vi "User Interface Global.vi"(6 "data2":variant, 7 "command (Update UI)":T2=enum."Update UI", 8 "error in":errorcluster, 9 "data1":variant, 10 "action":T1, 11 "user interface queue reference":T3) -> (0 "error out":errorcluster)   [LabVIEW 2011]
uses:
  Controls/User Interface Queue Reference.ctl
  Controls/User Interface Control.ctl
  Controls/User Interface Action.ctl
  User Interface Global.ctl
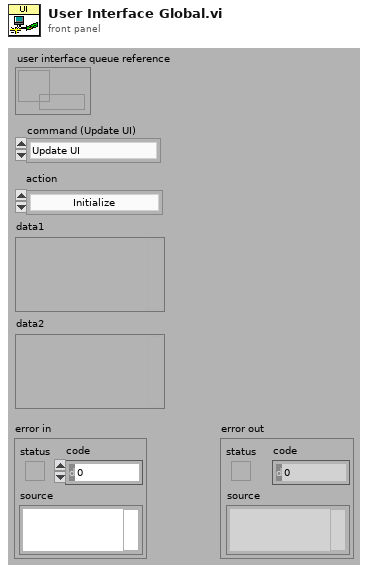
[diagram p1: front panel]
types:
  T1 = typedef "User Interface Action.ctl" = enum16{"Initialize", "Data Acquisition Disable", "Data View Disable", "Sample Set", "Sample Set 2D Data", "Sample Set x0 & dx", "Sample Add", "Sample Set Cursor", "Sample Set Offset & Multiplier", "Sample Set Axis Labels", "Sample Parameters Disabled", "Sample Parameters Update", "Run Update", "Run Set Offset & Multiplier", "Run Set Axis Labels", "Run Set Cursor", "Run Set Disabled", "Run Parameters Update", "Run Parameters Disabled", "Run Number Set", "Run Number Set Range", "Run Number Set Disabled", "Sample Number Set", "Sample Number Set Range", "Notes Set Value", "Update Plot", "Set Plot Parameters", "Update Concentration Plot", "Time Set", "Clear DAQ Display", "Clear Analysis Display", "Status Bar Set", "Progress Bar Set", "Display Mode Set", "Experiment Type Set", "Analysis Plot Average Set", "Stop"}
  T2 = typedef "User Interface Global.ctl" = enum16{"Initialize", "Update UI", "Stop"}
  T3 = typedef "User Interface Queue Reference.ctl" = refnum<queue>
  T4 = typedef "User Interface Control.ctl" = cluster{"action":T1, "data1":variant, "data2":variant}
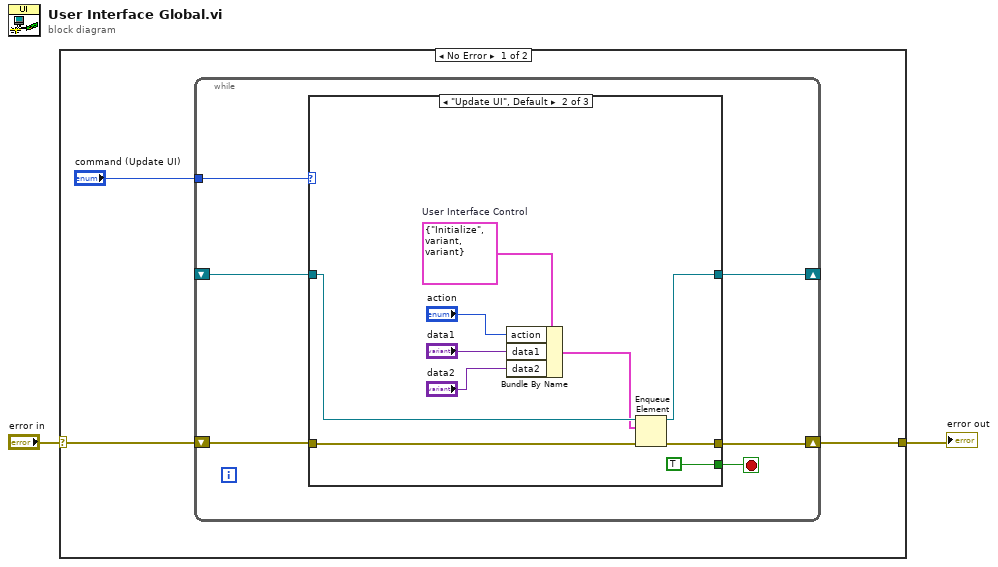
[diagram p0: block diagram]
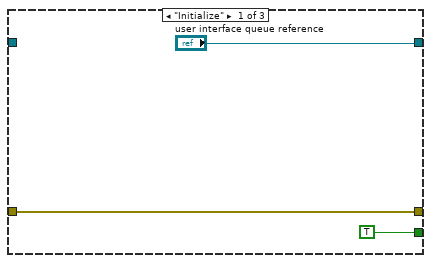
[diagram p2: hidden frame]
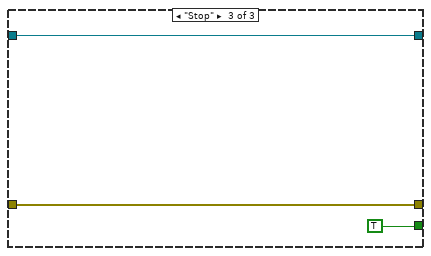
[diagram p3: hidden frame]
diagram:
  n1 = case shown="No Error" "error in" {
    selector: "error in" -> [w5 w28]
    tunnel: [w4 w28] -> w1
    frame No Error {
      n2 = while {
        shift-right: [w9] -> w4
        shift-left: w5 -> [w10]
        tunnel: "command (Update UI)" -> [w8]
        shift-right: [w7] -> _
        shift-left: _ -> [w6]
        stop <- w11 stop-if-true
        n3 = case shown="\"Update UI\", Default" w8 {
          tunnel: [TRUE TRUE TRUE] -> w11
          tunnel: w10 -> [w13 w22 w27]
          tunnel: [w13 w21 w27] -> w9
          tunnel: ["user interface queue reference" w18 w25] -> w7
          tunnel: w6 -> [_ w20 w25]
          frame "Initialize" {
          }
          frame "Update UI", Default {
            w17 = T4 {"action"=enum."Initialize", "data1"=variant, "data2"=variant}  # User Interface Control
            n4 = Bundle By Name(cluster=w17, "action"="action", "data1"="data1", "data2"="data2") -> (w19:T4)
            n5 = Enqueue Element(queue=w20, element=w19, error in (no error)=w22) -> (queue out=w18:T3, error out=w21:errorcluster)  [unwired: 1 in, 1 out]
          }
          frame "Stop" {
          }
        }
      }
    }
    frame Error {
    }
  }
  "error out" <- w1
